vi "i2c_delta_t_stats.vi"(5 "Input":T1[](array[typedef]), 11 "Threshold":u16=500) -> (6 "Results":cluster{"Min":u16, "Max":u16, "Mean":sgl}, 15 "Big delta t":i32[](array[numeric]))   [LabVIEW 2012]
uses:
  i2c_status_cluster.ctl
  Common/i2c_status.ctl
panel:
  # "Return indices where delta t is above this threshold."
  # "Extract statistics from the timestamp increments in status data."
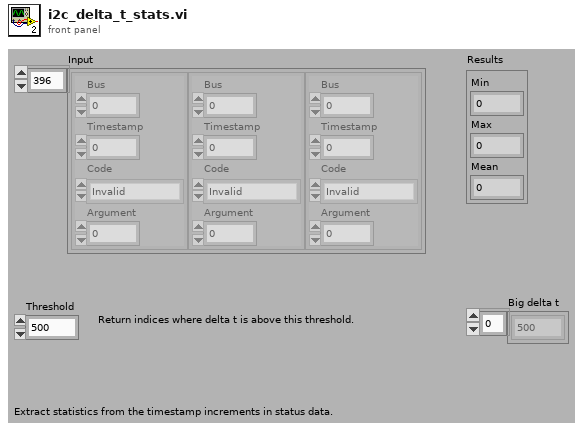
[diagram p1: front panel]
types:
  T1 = typedef "i2c_status_cluster.ctl" = cluster{"Bus":u8, "Timestamp":u16, "Code":T2, "Argument":u8}
  T2 = typedef "i2c_status.ctl" = enum8{"Invalid", "Command", "I2C start", "Trigger wait", "TX data wait", "Sequence", "Receive data", "I2C error", "Address NACK", "Data NACK", "SDA stuck", "SCL stuck", "Bad command"}
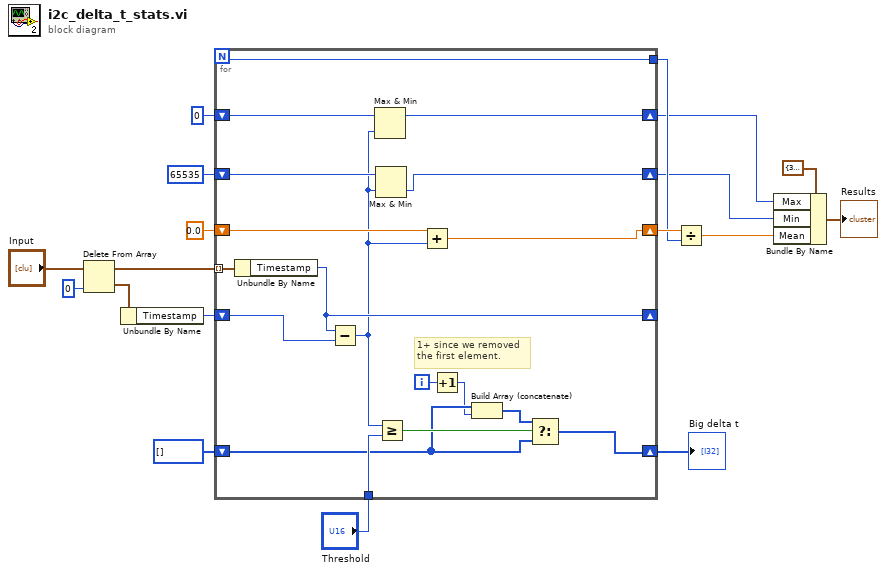
[diagram p0: block diagram]
diagram:
  n1 = Delete From Array(array="Input", index=0) -> (deleted portion=w10:T1, array with subset deleted=w9:T1[])  [unwired: 1 in]
  n2 = Unbundle By Name(w10) -> ("Timestamp"=w18:u16)
  n3 = for {
    N -> [w33]
    tunnel: w9 -> [w21] mode=indexing
    shift-right: [w35] -> _
    shift-left: w18 -> [w36]
    shift-right: [w30] -> w5
    shift-left: u16 65535 ("Timestamp") -> [w31]
    shift-right: [w32] -> w14
    shift-left: sgl 0.0 ("Timestamp") -> [w34]
    tunnel: [w33] -> w13
    shift-right: [w28] -> w6
    shift-left: u16 0 ("Timestamp") -> [w29]
    tunnel: "Threshold" -> [w27]
    shift-right: [w23] -> w1
    shift-left: i32[] [] -> [w25]
    i -> [w20]
    # "1+ since we removed\nthe first element."
    n4 = Unbundle By Name(w21) -> ("Timestamp"=w35:u16)
    n5 = Subtract(x=w35, y=w36) -> (x-y=w22:u16)
    n6 = Max & Min(x=w29, y=w22) -> (max(x,y)=w28:u16)  [unwired: 1 out]
    n7 = Max & Min(x=w31, y=w22) -> (min(x,y)=w30:u16)  [unwired: 1 out]
    n8 = Greater Or Equal?(x=w22, y=w27) -> (x >= y?=w26:bool)
    n9 = Add(x=w34, y=w22) -> (x+y=w32:sgl)
    n10 = Increment(x=w20) -> (x+1=w19:i32)
    n11 = Build Array (concatenate)(w25, w19) -> (w24:i32[])
    n12 = Select(t=w24, s=w26, f=w25) -> (s? t:f=w23:i32[])
  }
  "Big delta t" <- w1
  n13 = Divide(x=w14, y=w13) -> (x/y=w4:sgl)
  n14 = Bundle By Name(cluster=cluster{"Min":u16, "Max":u16, "Mean":sgl} {"Min"=367, "Max"=784, "Mean"=396.30908} ("Results"), "Max"=w6, "Min"=w5, "Mean"=w4) -> (→"Results":cluster{"Min":u16, "Max":u16, "Mean":sgl})
